vi "超标留样启动运行.vi"(8 "error in (no error)":errorcluster) -> (0 "error out":errorcluster)   [LabVIEW 2016, in "超标留样集成.lvlib" / "德润DR803M超标留样.lvlib"]
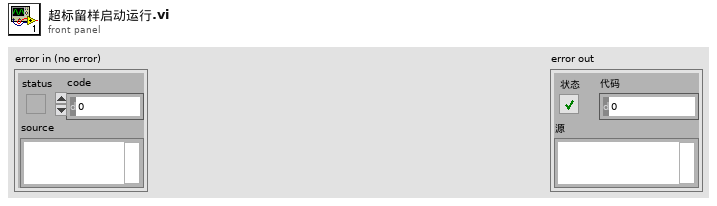
[diagram p1: front panel]
types:
  T1 = typedef "超标留样集成.lvlib/德润DR803M超标留样.lvlib/typedef.ctl" = cluster{"枚举":enum16{"open", "read", "write", "close", "write_register"}, "写入内容":string, "data_in":cluster{"write_coil_in":cluster{"address":u16, "value":bool}, "write_register_in":cluster{"address":u16, "values":u16[]}, "read_register_in":cluster{"starting address":u16, "quantity":u16}}}
  T2 = enum16{"open", "read", "write", "close", "write_register"}
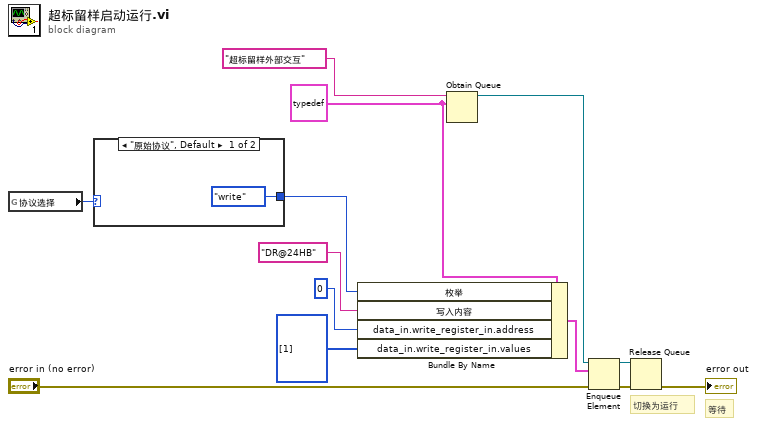
[diagram p0: block diagram]
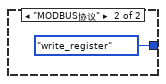
[diagram p2: hidden frame]
diagram:
  w5 = T1 {"枚举"=enum."open", "写入内容"="超标留样", "data_in"={"write_coil_in"={"address"=0, "value"=FALSE}, "write_register_in"={"address"=0, "values"=[]}, "read_register_in"={"starting address"=0, "quantity"=0}}}
  # "等待"
  # "切换为运行"
  n1 = global read "超标留样全局.vi" "协议选择"() -> (w4:enum16{"原始协议", "MODBUS协议"})
  n2 = case shown="\"原始协议\", Default" w4 {
    tunnel: [T2."write" ("枚举") T2."write_register" ("枚举")] -> w3
    frame "原始协议", Default {
    }
    frame "MODBUS协议" {
    }
  }
  n3 = Bundle By Name(cluster=w5, "枚举"=w3, "写入内容"="DR@24HB", "data_in.write_register_in.address"=u16 0, "data_in.write_register_in.values"=u16[] [1]) -> (w9:T1)
  n4 = Obtain Queue(name (unnamed)="超标留样外部交互" ("名称（未命名）"), element data type=w5) -> (queue out=w12:refnum<queue>)  [unwired: 3 in, 2 out]
  n5 = Enqueue Element(queue=w12, element=w9, error in (no error)="error in (no error)") -> (queue out=w7:refnum<queue>, error out=w8:errorcluster)  [unwired: 1 in, 1 out]
  n6 = Release Queue(queue=w7, error in (no error)=w8) -> (error out=→"error out":errorcluster)  [unwired: 1 in, 2 out]
